vi "test do.vi"() -> ()   [LabVIEW 2019]
panel:
  out "x != y?":bool
  out "output 1":i32
  out "Label.Text":string
  in  "DO 3":bool caption="Вода Y18.1 [DO3]"
  in  "DO 4":bool caption="Вода Y18.2 [DO4]"
  in  "DO 5":bool caption="KP6 Y29.1 33.7"
  in  "DO 0":bool caption="KP1 [DO 0]"
  in  "DO 2":bool caption="Пуск KP3 [DO 2]"
  in  "DO 6":bool caption="KP7 Y29.2 33.8"
  in  "DO 7":bool caption="KP8 Y29.3 33.9"
  in  "DO 8":bool caption="KP9 Y29.4  33.12"
  in  "DO 13":bool caption="KP14 Y29.9 33.10"
  in  "DO 9":bool caption="KP10 Y29.5 33.1"
  in  "DO 10":bool caption="KP11 Y29.6 33.2"
  in  "DO 11":bool caption="KP12 Y29.7  33.13"
  in  "DO 12":bool caption="KP13 Y29.8  33.11"
  in  "DO 14":bool caption="KP15 Y29.10  33.6"
  in  "DO 15":bool caption="KP16 Y29.11  33.5"
  in  "DO 16":bool caption="KP17 Y29.12  33.4"
  in  "DO 1":bool caption="Пуск KP2 [DO 1]"
  in  "DO 18":bool caption="Подача воздук KP19"
  in  "DO 17":bool caption="KP18 Y29.13 33.3"
  in  "DO 19":bool caption="Драйверы KP20"
  in  "DO 20":bool caption="KP21 Y44.1 ОТК."
  in  "DO 21":bool caption="KP22 Y44.1 抢市."
  in  "DO 23":bool caption="KP24 Y44.2 抢市."
  in  "DO 22":bool caption="KP23 Y44.2 ОТК."
  in  "DO 24":bool caption="Stop SD 1"
  in  "DO 25":bool caption="Stop SD 2 [37.1]"
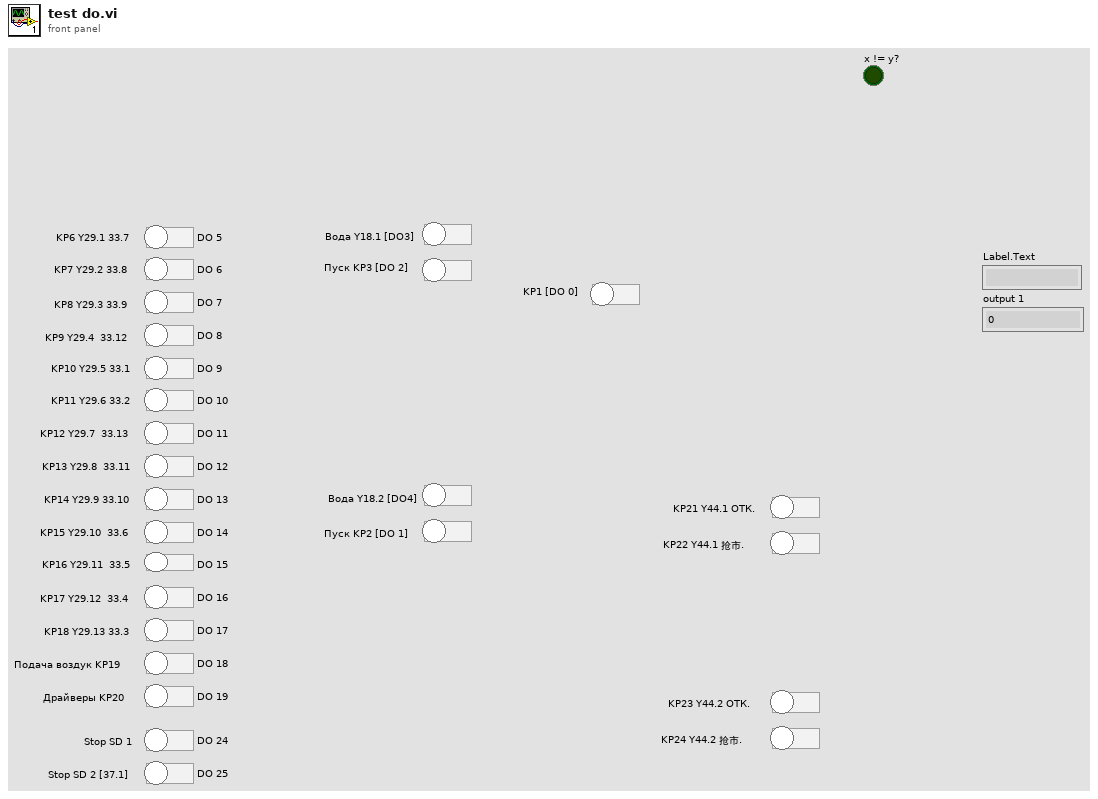
[diagram p1: front panel]
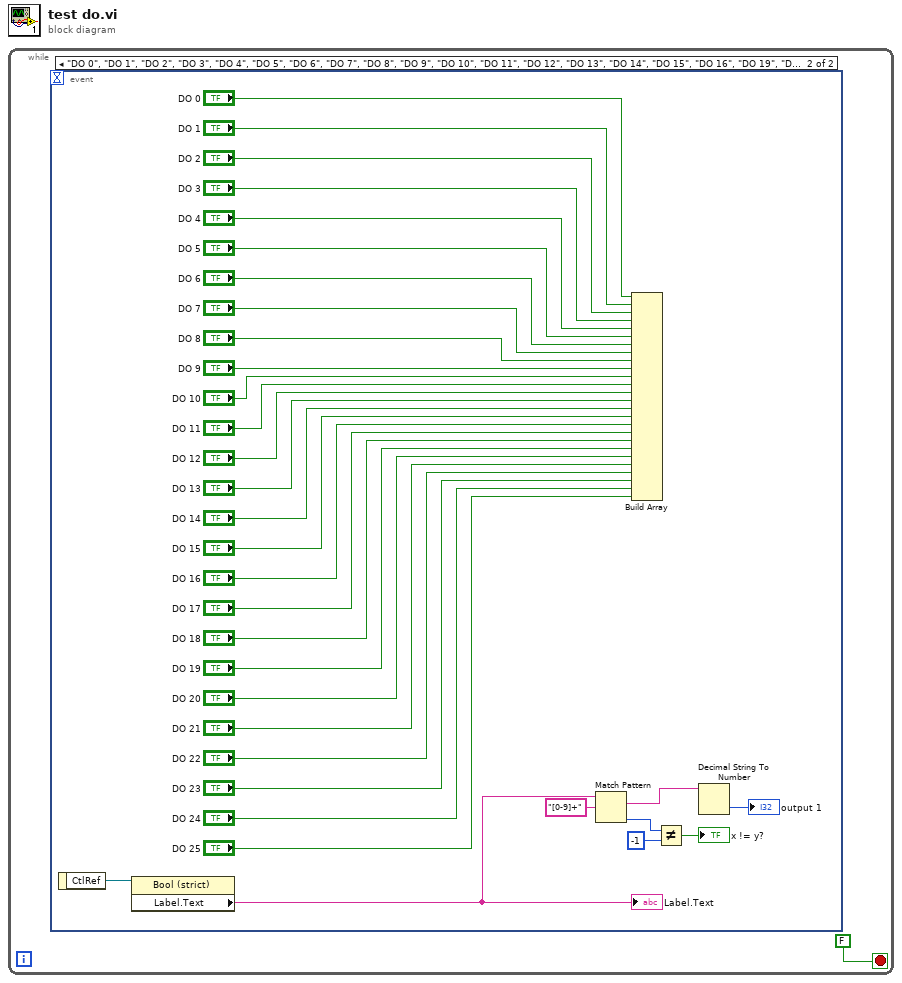
[diagram p0: block diagram]
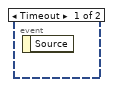
[diagram p2: hidden frame]
diagram:
  n1 = while {
    stop <- FALSE stop-if-true
    n2 = event shown="[1] \"DO 0\", \"DO 1\", \"DO 2\", \"DO 3\", \"DO 4\", \"DO 5\", \"DO 6\", \"DO 7\", \"DO 8\", \"DO 9\", \"DO 10\", \"DO 11\", \"DO 12\", \"DO 13\", \"DO 14\", \"DO 15\", \"DO 16\", \"DO 19\", \"DO 17\", \"DO 18\", \"DO 20\", \"DO 21\", \"DO 22\", \"DO 23\", \"DO 24\", \"DO 25\": Value Change" {
      selector: _ -> [_ _]
      dyn-events: _ -> [_ _]
      timeout: _ -> [_ _]
      event Timeout {
        n3 = event-data() -> ()  [unwired: 1 in, 1 out]
      }
      event "DO 0", "DO 1", "DO 2", "DO 3", "DO 4", "DO 5", "DO 6", "DO 7", "DO 8", "DO 9", "DO 10", "DO 11", "DO 12", "DO 13", "DO 14", "DO 15", "DO 16", "DO 19", "DO 17", "DO 18", "DO 20", "DO 21", "DO 22", "DO 23", "DO 24", "DO 25": Value Change {
        n4 = event-data() -> ("CtlRef"=w9:refnum<vi>)  [unwired: 1 in]
        n5 = property class="Bool (strict)"(reference=w9) -> ("Label.Text"=w3:string)  [unwired: 1 in, 2 out]
        "Label.Text" <- w3
        n6 = Match Pattern(string=w3, regular expression="[0-9]+") -> (match substring=w5:string, offset past match=w7:i32)  [unwired: 1 in, 2 out]
        n7 = Build Array("DO 0", "DO 1", "DO 2", "DO 3", "DO 4", "DO 5", "DO 6", "DO 7", "DO 8", "DO 9", "DO 10", "DO 11", "DO 12", "DO 13", "DO 14", "DO 15", "DO 16", "DO 17", "DO 18", "DO 19", "DO 20", "DO 21", "DO 22", "DO 23", "DO 24", "DO 25") -> ()  [unwired: 1 out]
        n8 = Not Equal?(x=w7, y=-1) -> (x != y?=→"x != y?":bool)
        n9 = Decimal String To Number(string=w5) -> (number=→"output 1":i32)  [unwired: 2 in, 1 out]
      }
    }
  }
